vi "FrontPanel.DeferPanelUpdates.vi"(8 "error in":errorcluster, 10 "Defer Panel Updates":bool=TRUE) -> (0 "error out":errorcluster)   [LabVIEW 2019, in "Tools.lvlib"]
uses:
  Tools.lvlib
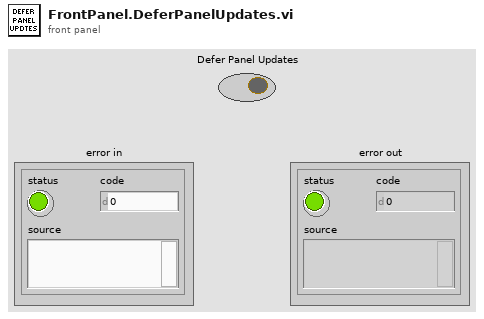
[diagram p1: front panel]
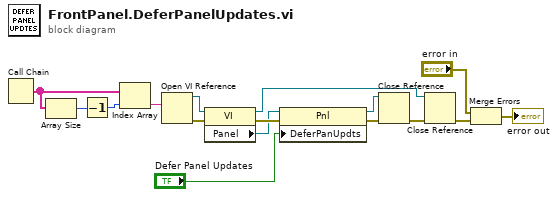
[diagram p0: block diagram]
diagram:
  n1 = Call Chain() -> (call chain=w11:string[])
  n2 = Array Size(array=w11) -> (size(s)=w12:i32)
  n3 = Decrement(x=w12) -> (x-1=w13:i32)
  n4 = Index Array(array=w11, index=w13) -> (element=w14:string)
  n5 = Open VI Reference(vi path=w14) -> (vi reference=w15:refnum<vi>, error out=w16:errorcluster)  [unwired: 5 in]
  n6 = property class="VI"(reference=w15, error in=w16) -> (reference out=w3:refnum<vi>, error out=w10:errorcluster, "Panel"=w8:refnum<vi>)
  n7 = property class="Pnl"(reference=w8, error in=w10, "DeferPanUpdts"="Defer Panel Updates") -> (reference out=w4:refnum<vi>, error out=w7:errorcluster)
  n8 = Close Reference(reference=w4, error in (no error)=w7) -> (error out=w6:errorcluster)
  n9 = Close Reference(reference=w3, error in (no error)=w6) -> (error out=w5:errorcluster)
  n10 = Merge Errors("error in", w5) -> (→"error out":errorcluster)
